vi "Get Instrument Alias.vi"(8 "error in (no error)":errorcluster, 11 "Instrument Control Board in":refnum<class "Instrument Control Board.lvclass">) -> (0 "error out":errorcluster, 2 "Instrument Alias":string, 3 "Instrument Control Board out":refnum<class "Instrument Control Board.lvclass">)   [LabVIEW 2023, in "HAF.lvlib" / "Instrument Control Board.lvclass"]
doc: "Returns the alias name of the Instrument for this Driver that can be used to initiate a session. Must be implemented by Subclasses because there is no Visa Session available to obtain it from when it is needed.\n\nIt's not ideal: need to think of a better way of dealing with attached resources than hard-coded aliases which must match what was entered in NI-MAX."
uses:
  Instrument Control Board.lvclass
  Instrument Control Board.lvclass/Instrument Control Board.ctl
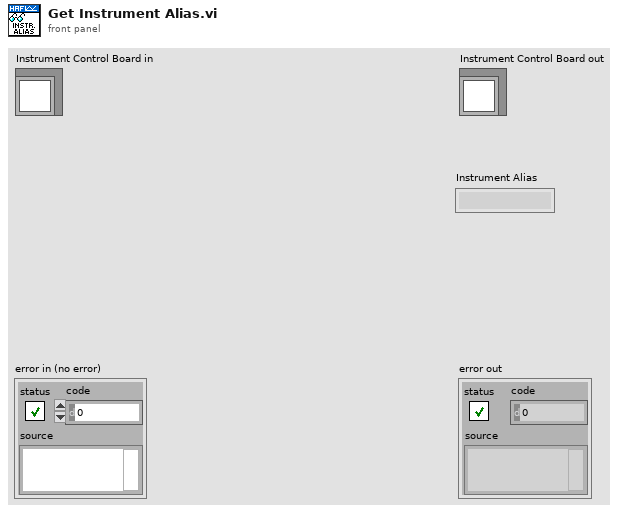
[diagram p1: front panel]
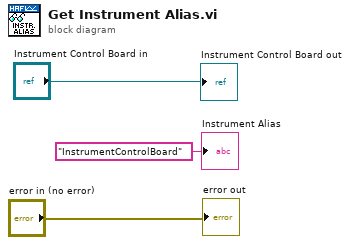
[diagram p0: block diagram]
diagram:
  "error out" <- "error in (no error)"
  "Instrument Control Board out" <- "Instrument Control Board in"
  "Instrument Alias" <- "InstrumentControlBoard" ("Instrument Alias")
